vi "Draw Estimated Pose.vi"(10 "Radius":dbl=1.0, 11 "State":T1) -> (3 "Estimated Pose":cluster{dbl[], dbl[]}(graph))   [LabVIEW 2020]
uses:
  <vilib>/Analysis/Matrix/Datatypes/RealMatrix.ctl
  <vilib>/Analysis/baseanly.llb/Real A x B.vi
  <vilib>/Analysis/Matrix/NI_Matrix.lvlib
  <vilib>/Analysis/NI_AALBase.lvlib
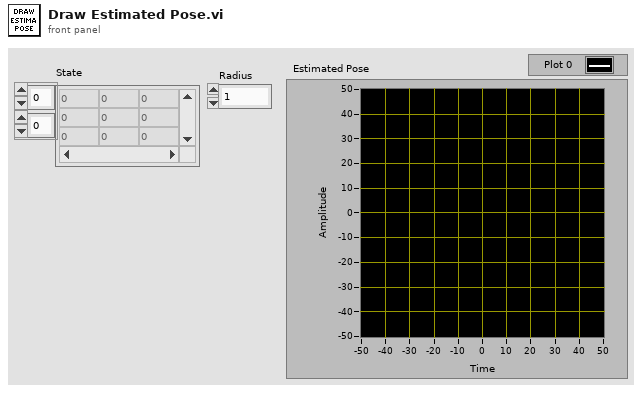
[diagram p1: front panel]
types:
  T1 = typedef "NI_Matrix.lvlib/RealMatrix.ctl" = dbl[][]
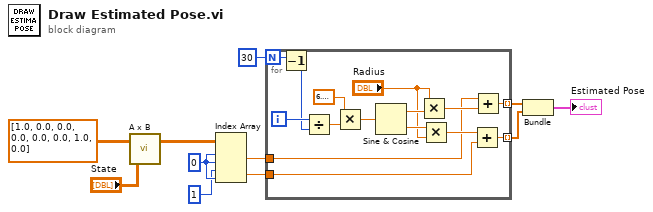
[diagram p0: block diagram]
diagram:
  w7 = 0 ("disabled index (col)")
  n1 = call-poly <vilib>:"A x B.vi"("B"="State", "A"=T1 [[1.0, 0.0, 0.0, 0.0], [0.0, 0.0, 1.0, 0.0]] ("Initial Control Input")) -> ("A x B"=w8:T1)  [unwired: 1 out]
  n2 = Index Array(array=w8, index (row) #1=w7, index (col) #1=w7, index (row) #2=1 ("index (col)"), index (col) #2=w7) -> (element #1=w10:dbl, element #2=w9:dbl)
  n3 = for {
    N: 30 -> [w13]
    tunnel: w9 -> [w17]
    tunnel: w10 -> [w18]
    tunnel: [w16] -> w4 mode=indexing
    tunnel: [w15] -> w3 mode=indexing
    i -> [w26]
    n4 = Decrement(x=w13) -> (x-1=w12:i32)
    n5 = Divide(x=w26, y=w12) -> (x/y=w25:dbl)
    n6 = Multiply(x=6.283185307179586, y=w25) -> (x*y=w23:dbl)
    n7 = Sine & Cosine(0:w23) -> (1:w22:dbl, 2:w21:dbl)
    n8 = Multiply(x="Radius", y=w22) -> (x*y=w20:dbl)
    n9 = Multiply(x=w21, y="Radius") -> (x*y=w19:dbl)
    n10 = Add(x=w19, y=w17) -> (x+y=w15:dbl)
    n11 = Add(x=w18, y=w20) -> (x+y=w16:dbl)
  }
  n12 = Bundle(w4, w3) -> (→"Estimated Pose":cluster{dbl[], dbl[]})  [unwired: 1 in]
